vi "waitx.vi"(1 "timeoutms":u32=120000, 2 "String Value":string(combo), 3 "连接ID":refnum<k5>) -> (0 "连接ID 2":refnum<k5>)   [LabVIEW 2017]
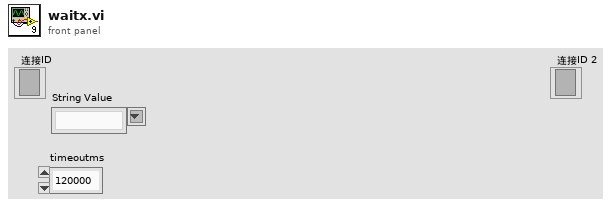
[diagram p1: front panel]
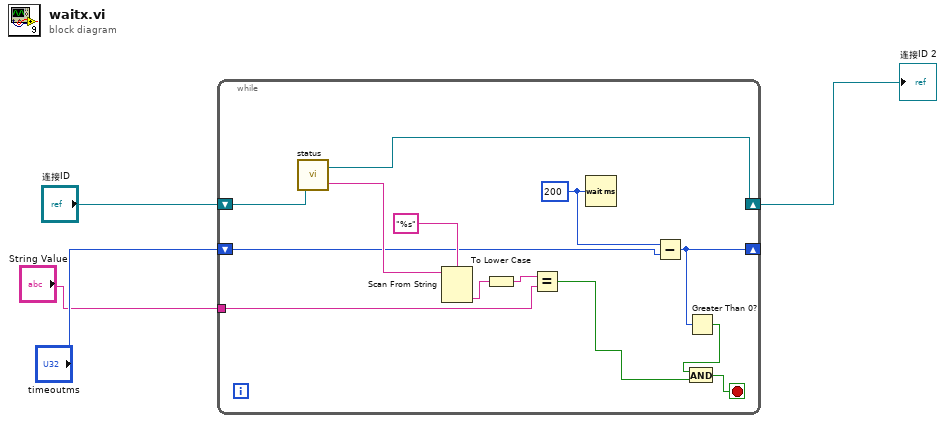
[diagram p0: block diagram]
diagram:
  n1 = while {
    shift-right: [w16] -> w1
    shift-left: "连接ID" -> [w17]
    shift-right: [w9] -> _
    shift-left: "timeoutms" -> [w10]
    tunnel: "String Value" -> [w5]
    stop <- w6 stop-if-true
    w11 = u32 200 ("等待时间（毫秒）")
    n2 = call "status.vi"("连接ID"=w17) -> ("连接ID输出"=w16:refnum<k5>, "String Value"=w15:string)
    n3 = Scan From String(format string="%s" ("格式字符串"), input string=w15) -> (output 1=w13:string)  [unwired: 3 in, 3 out]
    n4 = To Lower Case(string=w13) -> (all lower case string=w12:string)
    n5 = Equal?(x=w12, y=w5) -> (x = y?=w7:bool)
    n6 = Wait (ms)(milliseconds to wait=w11) -> ()  [unwired: 1 out]
    n7 = Subtract(x=w11, y=w10) -> (x-y=w9:u32)
    n8 = Greater Than 0?(x=w9) -> (x > 0?=w8:bool)
    n9 = And(x=w8, y=w7) -> (x .and. y?=w6:bool)
  }
  "连接ID 2" <- w1
